vi "Workshop Exercise 3 Solution.vi"() -> ()   [LabVIEW 2019]
panel:
  in  "Stop":bool
  out "Plot":cluster{dbl, dbl}(graph)
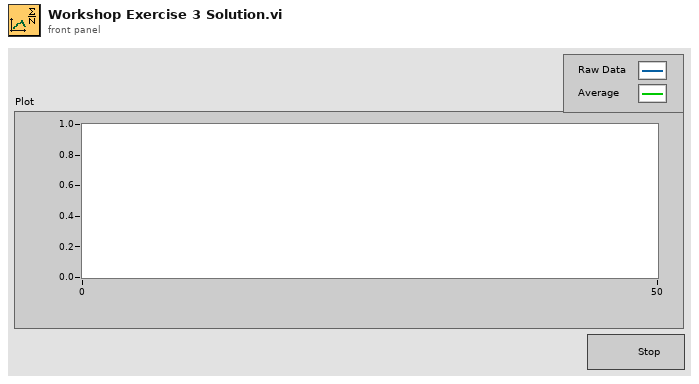
[diagram p1: front panel]
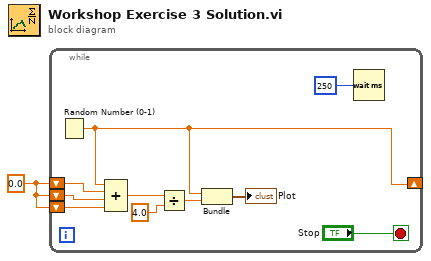
[diagram p0: block diagram]
diagram:
  w1 = 0.0
  n1 = while {
    shift-left: w1 -> [w7]
    shift-left: w1 -> [w6]
    shift-left: w1 -> [w5]
    shift-right: [w4] -> _
    stop <- "Stop" stop-if-true
    # "Plot Random Number and Running Average"
    n2 = Random Number (0-1)() -> (number: 0 to 1=w4:dbl)
    n3 = Compound Arithmetic op=ADD(w4, w5, w6, w7) -> (w3:dbl)
    n4 = Divide(x=w3, y=4.0) -> (x/y=w10:dbl)
    n5 = Bundle(w4, w10) -> (→"Plot":cluster{dbl, dbl})  [unwired: 1 in]
    n6 = Wait (ms)(milliseconds to wait=u32 250) -> ()  [unwired: 1 out]
  }
